vi "D2SParser - Private - Helper - Read Quad.vi"(8 "error in (no error)":errorcluster, 10 "Position":i64, 11 "D2SParser in":refnum<class "D2SParser.lvclass">) -> (0 "error out":errorcluster, 2 "quad":u64, 3 "D2SParser out":refnum<class "D2SParser.lvclass">)   [LabVIEW 2015, in "D2SParser.lvclass"]
uses:
  D2SParser.lvclass
  D2SParser.lvclass/D2SParser.ctl
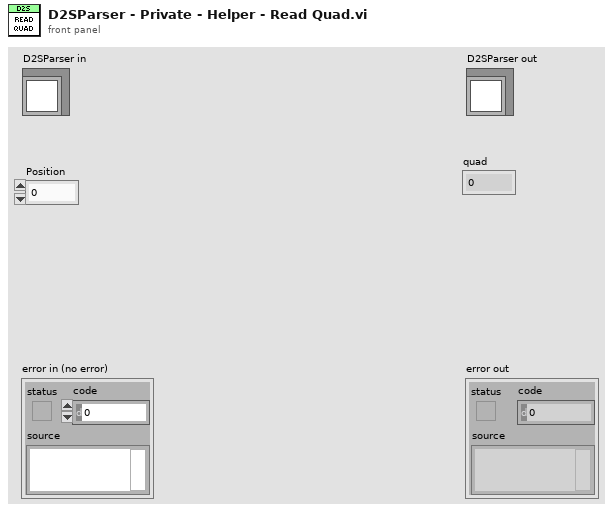
[diagram p1: front panel]
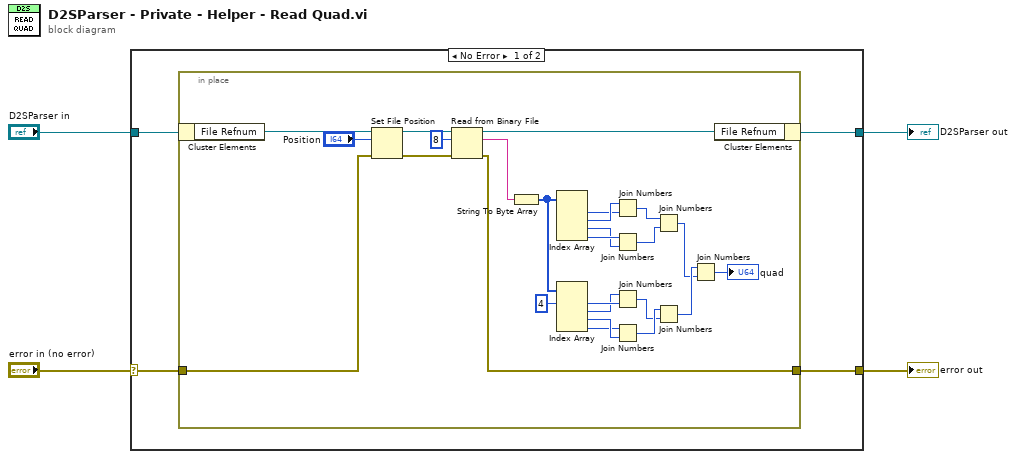
[diagram p0: block diagram]
diagram:
  n1 = case shown="No Error" "error in (no error)" {
    selector: "error in (no error)" -> [w7 w36]
    tunnel: [w6 w36] -> w3
    tunnel: [w5 w35] -> w1
    tunnel: "D2SParser in" -> [w8 w35]
    frame No Error {
      n2 = in-place {
        in-place-border: w7 -> [w29]
        in-place-border: [w27] -> w6
        n3 = in-place-cluster #1(w8) -> ("File Refnum"=w31:refnum<file>)
        n4 = Set File Position(offset (in bytes) (0)="Position", refnum=w31, error in=w29) -> (refnum out=w32:refnum<file>, error out=w33:errorcluster)  [unwired: 1 in]
        n5 = Read from Binary File(8:w33, 10:8 ("count (1)"), 11:w32) -> (0:w27:errorcluster, 2:w26:string, 3:w30:refnum<file>)  [unwired: 3 in, 1 out]
        n6 = String To Byte Array(string=w26) -> (unsigned byte array=w13:u8[])
        n7 = Index Array(array=w13) -> (element #1=w24:u8, element #2=w25:u8, element #3=w22:u8, element #4=w23:u8)  [unwired: 4 in]
        n8 = Index Array(array=w13, index #1=4 ("index")) -> (element #1=w15:u8, element #2=w14:u8, element #3=w17:u8, element #4=w16:u8)  [unwired: 3 in]
        n9 = Join Numbers(hi=w25, lo=w24) -> ((hi.lo)=w21:u16)
        n10 = Join Numbers(hi=w23, lo=w22) -> ((hi.lo)=w20:u16)
        n11 = Join Numbers(hi=w14, lo=w15) -> ((hi.lo)=w18:u16)
        n12 = Join Numbers(hi=w16, lo=w17) -> ((hi.lo)=w19:u16)
        n13 = Join Numbers(hi=w21, lo=w20) -> ((hi.lo)=w10:u32)
        n14 = Join Numbers(hi=w19, lo=w18) -> ((hi.lo)=w11:u32)
        n15 = Join Numbers(hi=w11, lo=w10) -> ((hi.lo)=→"quad":u64)
        n16 = in-place-cluster #1("File Refnum"=w30) -> (w5:refnum<class "D2SParser.lvclass">)
      }
    }
    frame Error {
    }
  }
  "error out" <- w3
  "D2SParser out" <- w1
